vi "Read Rescale Configuration.vi"(8 "error in (no error)":errorcluster, 11 "Rescale in":refnum<class "Rescale.lvclass">) -> (0 "error out":errorcluster, 2 "Configuration":T1, 3 "Rescale out":refnum<class "Rescale.lvclass">)   [LabVIEW 2018, in "Rescale.lvclass"]
uses:
  Rescale.lvclass
  C:/github/LabActor/Template Module/Template Module.lvclass
  Rescale Configuration.ctl
  NHMFL_Core/Libraries/File/Controls/NXG TDMS channel re-scale selector entry.ctl
  Template Module/Template Module.lvclass/Template Module.ctl
  Template Module/Read Configuration.vi
panel:
  # "Use   Group                     Channel                               New channel                                Scale"
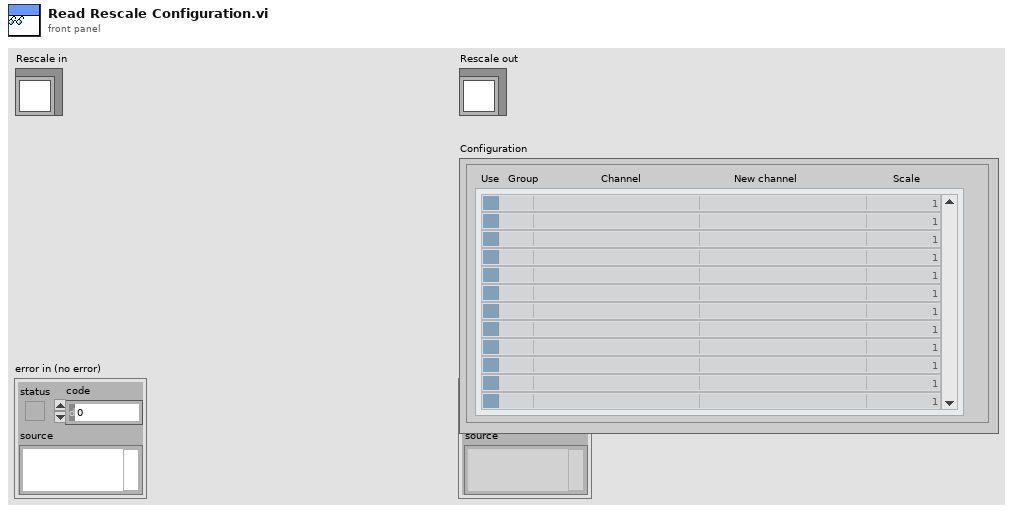
[diagram p1: front panel]
types:
  T1 = typedef "Rescale Configuration.ctl" = cluster{"Channels":T2[]}
  T2 = typedef "NXG TDMS channel re-scale selector entry.ctl" = cluster{"Group":string, "Channel":string, "Active":bool, "New channel":string, "Re-scale factor":dbl}
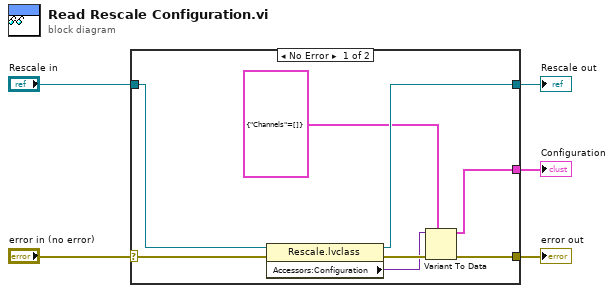
[diagram p0: block diagram]
diagram:
  n1 = case shown="No Error" "error in (no error)" {
    selector: "error in (no error)" -> [w13 w14]
    tunnel: [w9 w14] -> w4
    tunnel: [w10 w15] -> w2
    tunnel: "Rescale in" -> [w11 w15]
    tunnel: [w6 _] -> w1
    frame No Error {
      n2 = property class="Rescale.lvclass"(reference=w11, error in=w13) -> (reference out=w10:refnum<class "Rescale.lvclass">, error out=w12:errorcluster, "Accessors:Configuration"=w7:variant)
      n3 = Variant To Data(error in=w12, type=T1 {"Channels"=[]} ("Configuration"), Variant=w7) -> (data=w6:T1, error out=w9:errorcluster)
    }
    frame Error {
    }
  }
  "error out" <- w4
  "Rescale out" <- w2
  "Configuration" <- w1
